vi "TOPAZ.vi"(2 "stop":bool, 4 "wait":u32=250, 6 "Отправить команду":bool, 8 "Ослабление, дБ":ext format="%.2g", 9 "Длина волны, нм":enum16{"850", "1300", "1310", "1550"}(ring), 10 "Выбор команды:":T2(ring), 11 "COM-порт":refnum<visa-resource-name>="COM7") -> (3 "Ответ устройства:":string, 5 "прочитано":u32, 7 "отправлено":u32)   [LabVIEW 2018]
uses:
  <vilib>/Instr/_visa.llb/VISA Configure Serial Port (Instr).vi
panel:
  in  "Tab Control":T1(tab)
  # "Задание параметров:"
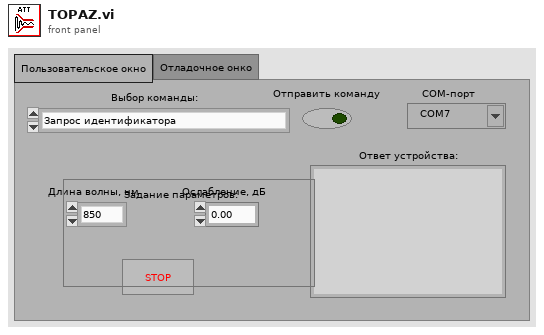
[diagram p1: front panel]
types:
  T1 = enum32{"Пользовательское окно", "Отладочное онко"}
  T2 = enum16{"Запрос идентификатора", "Запрос доступных длин волн, (нм)", "Запрос установленной длины волны, (нм)", "Запрос установленного ослабления, (дБ)", "Установка длины волны, (нм)", "Установка ослабления, (дБ)"}
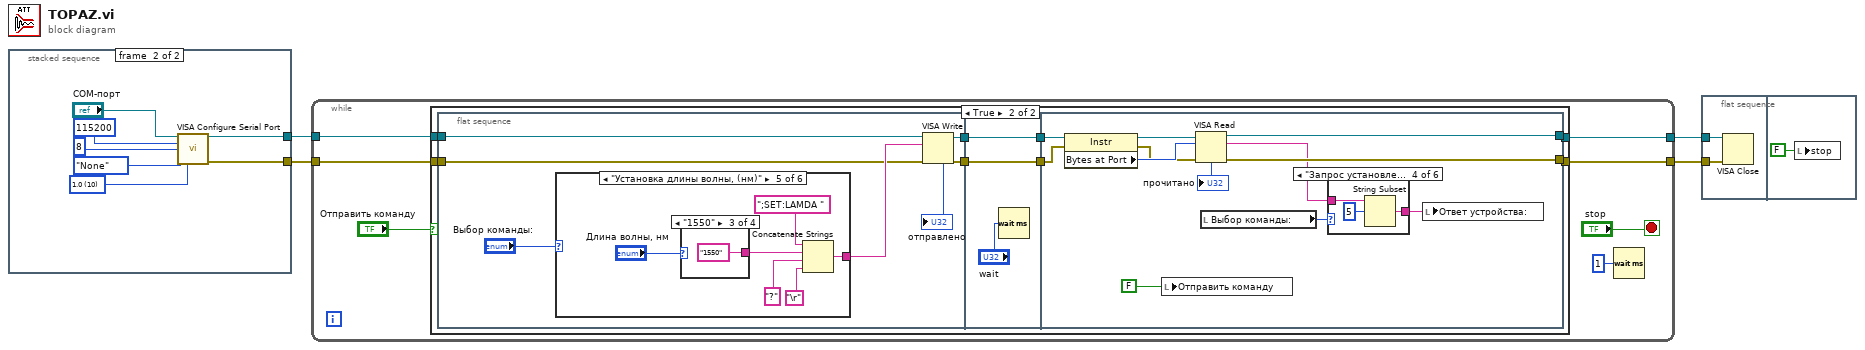
[diagram p0: block diagram]
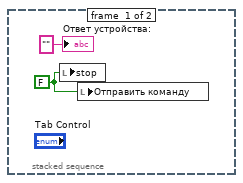
[diagram p2: hidden frame]
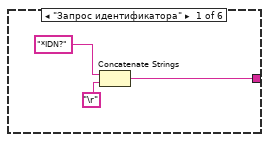
[diagram p4: hidden frame]
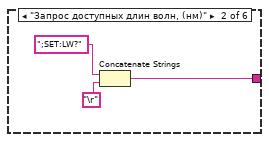
[diagram p5: hidden frame]
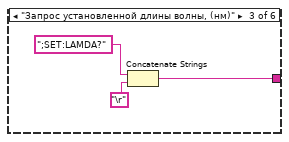
[diagram p6: hidden frame]
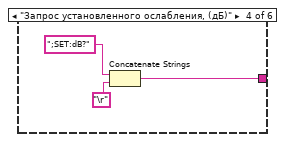
[diagram p7: hidden frame]
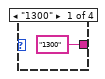
[diagram p8: hidden frame]
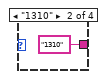
[diagram p9: hidden frame]
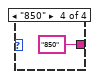
[diagram p10: hidden frame]
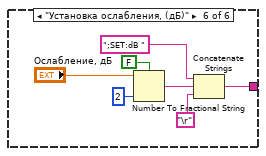
[diagram p11: hidden frame]
diagram:
  n1 = stacked-sequence {
    tunnel: [_ w8] -> w2
    tunnel: [_ w7] -> w1
    frame #0 {
      w5 = FALSE ("Текущее\nослабление? (дБ)")
      n2 = local write "stop"(w5) -> ()
      n3 = local write "Отправить команду"(w5) -> ()
      "Ответ устройства:" <- "" ("Ответ:")
    }
    frame #1 {
      w10 = u16 10 items=["1.0"=10, "1.5"=15, "2.0"=20] ("stop bits (10: 1 bit)")
      n4 = call-poly "VISA Configure Serial Port"("VISA resource name"="COM-порт", "baud rate (9600)"=u32 115200, "data bits (8)"=u16 8, "parity (0:none)"=enum16{"None", "Odd", "Even", "Mark", "Space"}."None", "stop bits (10: 1 bit)"=w10) -> ("VISA resource name out"=w8:refnum<visa-resource-name>, "error out"=w7:errorcluster)  [unwired: 9 in]
    }
  }
  n5 = while {
    tunnel: [w18] -> w4
    tunnel: [w17] -> w3
    tunnel: w2 -> [w16]
    tunnel: w1 -> [w15]
    stop <- "stop" stop-if-true
    n6 = case shown="True" "Отправить команду" {
      tunnel: [w22 w28] -> w18
      tunnel: [w21 w25] -> w17
      tunnel: w16 -> [w22 w24]
      tunnel: w15 -> [w21 w23]
      frame False {
      }
      frame True {
        n7 = flat-sequence {
          tunnel: [w37] -> w29
          tunnel: [w35] -> w26
          tunnel: w24 -> [w34]
          tunnel: w23 -> [w31]
          tunnel: [w69] -> w30
          tunnel: w29 -> [w69]
          tunnel: [w68] -> w27
          tunnel: w26 -> [w68]
          tunnel: w30 -> [w79]
          tunnel: [w75] -> w28
          tunnel: w27 -> [w77]
          tunnel: [w74] -> w25
          frame #0 {
            n8 = case shown="\"Установка длины волны, (нм)\"" "Выбор команды:" {
              tunnel: [w38 w41 w44 w47 w50 w60] -> w32
              frame "Запрос идентификатора" {
                n9 = Concatenate Strings("*IDN?", "\r") -> (w38:string)
              }
              frame "Запрос доступных длин волн, (нм)" {
                n10 = Concatenate Strings(";SET:LW?", "\r") -> (w41:string)
              }
              frame "Запрос установленной длины волны, (нм)" {
                n11 = Concatenate Strings(";SET:LAMDA?", "\r") -> (w44:string)
              }
              frame "Запрос установленного ослабления, (дБ)" {
                n12 = Concatenate Strings(";SET:dB?", "\r") -> (w47:string)
              }
              frame "Установка длины волны, (нм)" {
                n13 = case shown="\"1550\"" "Длина волны, нм" {
                  tunnel: ["1300" "1310" "1550" "850"] -> w51
                  frame "1300" {
                  }
                  frame "1310" {
                  }
                  frame "1550" {
                  }
                  frame "850" {
                  }
                }
                n14 = Concatenate Strings(";SET:LAMDA ", w51, "?" ("string"), "\r") -> (w50:string)
              }
              frame "Установка ослабления, (дБ)" {
                n15 = Number To Fractional String(use system decimal point (T)=FALSE, number="Ослабление, дБ", precision (6)=i16 2) -> (F-format string=w64:string)  [unwired: 1 in]
                n16 = Concatenate Strings(";SET:dB ", w64, "\r") -> (w60:string)
              }
            }
            n17 = VISA Write(VISA resource name=w34, write buffer=w32, error in (no error)=w31) -> (VISA resource name out=w37:refnum<visa-resource-name>, return count=→"отправлено":u32, error out=w35:errorcluster)
          }
          frame #1 {
            n18 = Wait (ms)(milliseconds to wait="wait") -> ()  [unwired: 1 out]
          }
          frame #2 {
            n19 = property class="Instr"(reference=w79, error in=w77) -> (reference out=w80:refnum<visa-resource-name>, error out=w73:errorcluster, "Bytes at Port"=w76:u32)
            n20 = local write "Отправить команду"(FALSE ("Текущее\nослабление? (дБ)")) -> ()
            n21 = VISA Read(VISA resource name=w80, byte count=w76, error in (no error)=w73) -> (VISA resource name out=w75:refnum<visa-resource-name>, read buffer=w71:string, return count=→"прочитано":u32, error out=w74:errorcluster)
            n22 = local read "Выбор команды:"() -> (w72:T2)
            n23 = case shown="\"Запрос установленного ослабления, (дБ)\"" w72 {
              tunnel: w71 -> [w82 w83 w84 w86 w88 w89]
              tunnel: [w82 w83 w84 w85 w88 w89] -> w70
              frame "Запрос идентификатора", Default {
              }
              frame "Запрос доступных длин волн, (нм)" {
              }
              frame "Запрос установленной длины волны, (нм)" {
              }
              frame "Запрос установленного ослабления, (дБ)" {
                n24 = String Subset(string=w86, offset (0)=5) -> (substring=w85:string)  [unwired: 1 in]
              }
              frame "Установка длины волны, (нм)" {
              }
              frame "Установка ослабления, (дБ)" {
              }
            }
            n25 = local write "Ответ устройства:"(w70) -> ()
          }
        }
      }
    }
    n26 = Wait (ms)(milliseconds to wait=u32 1) -> ()  [unwired: 1 out]
  }
  n27 = flat-sequence {
    tunnel: w4 -> [w91]
    tunnel: w3 -> [w90]
    frame #0 {
      n28 = VISA Close(VISA resource name=w91, error in (no error)=w90) -> ()  [unwired: 1 out]
    }
    frame #1 {
      n29 = local write "stop"(FALSE ("stop")) -> ()
    }
  }
